vi "Position Right Vertical Splitter.vi"(8 "error in (no error)":errorcluster, 10 "Splitter Position":i32, 11 "This VI":refnum<vi>) -> (0 "error out":errorcluster)   [LabVIEW 2014]
uses:
  <vilib>/Utility/miscctls.llb/LVPointTypeDef.ctl
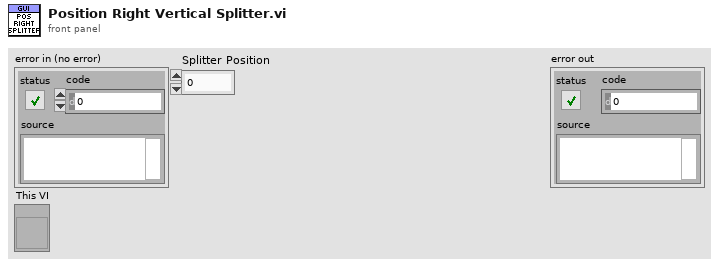
[diagram p1: front panel]
types:
  T1 = typedef "LVPointTypeDef.ctl" = cluster{"Horizontal":i16, "Vertical":i16}
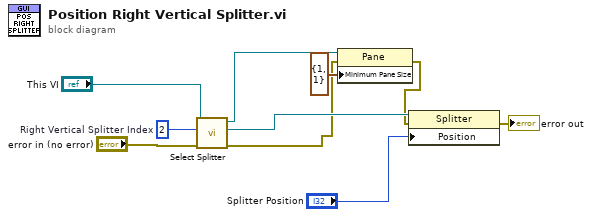
[diagram p0: block diagram]
diagram:
  w8 = 2  # Right Vertical Splitter Index
  n1 = call "Select Splitter.vi"("error in (no error)"="error in (no error)", "Pane Index"=w8, "This VI"="This VI") -> ("error out"=w1:errorcluster, "Splitter"=w7:refnum<vi>, "Pane"=w4:refnum<vi>)  [unwired: 6 in]
  n2 = property class="Pane"(reference=w4, error in=w1, "Minimum Pane Size"=T1 {"Horizontal"=1, "Vertical"=1}) -> (error out=w2:errorcluster)  [unwired: 1 out]
  n3 = property class="Splitter"(reference=w7, error in=w2, "Position"="Splitter Position") -> (error out=→"error out":errorcluster)  [unwired: 1 out]
